vi "Load Action Core.vi"(8 "error in (no error)":errorcluster, 10 "config file in":T1, 11 "NI DMM in":refnum<class "NI DMM.lvclass">) -> (0 "error out":errorcluster, 2 "config file out":T1, 3 "NI DMM out":refnum<class "NI DMM.lvclass">)   [LabVIEW 2023, in "NI DMM.lvlib" / "NI DMM.lvclass"]
uses:
  NI DMM.lvclass
  <vilib>/Utility/config.llb/Config Data RefNum.ctl
  NI DMM.lvclass/NI DMM.ctl
  <vilib>/Utility/config.llb/NI_LVConfig.lvlib
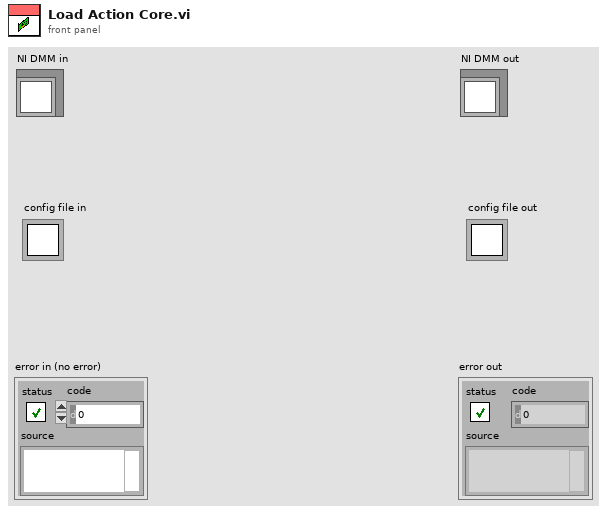
[diagram p1: front panel]
types:
  T1 = typedef "NI_LVConfig.lvlib/Config Data RefNum.ctl" = refnum<k1>
  T2 = cluster{"instrument_descriptor":refnum<k15>, "function":i32, "sampling_rate":dbl, "number_to_fetch":i32, "range":dbl}
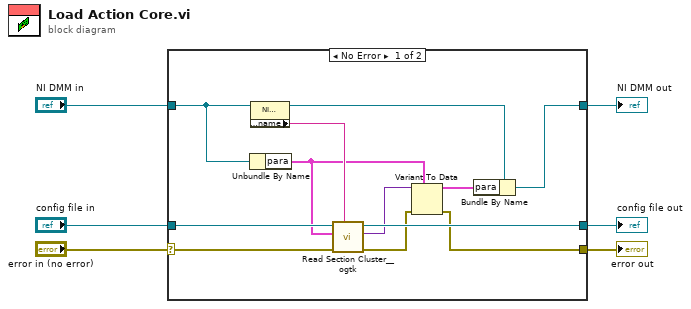
[diagram p0: block diagram]
diagram:
  n1 = case shown="No Error" "error in (no error)" {
    selector: "error in (no error)" -> [w18 w21]
    tunnel: [w12 w21] -> w5
    tunnel: "config file in" -> [w15 w20]
    tunnel: "NI DMM in" -> [w17 w19]
    tunnel: [w14 w20] -> w2
    tunnel: [w7 w19] -> w1
    frame No Error {
      n2 = Unbundle By Name(w17) -> ("para"=w11:T2)
      n3 = property class="NI DMM.lvclass"(reference=w17) -> (reference out=w9:refnum<class "NI DMM.lvclass">, "Accessor:name"=w16:string)  [unwired: 1 in, 1 out]
      n4 = call <userlib>:"Read Section Cluster__ogtk.vi"("section (optional)"=w16, "error in (no error)"=w18, "Section Formatted Cluster Type"=w11, "refnum"=w15) -> ("error out"=w13:errorcluster, "Section Formatted Cluster"=w10:variant, "dup refnum"=w14:T1)  [unwired: 3 in, 2 out]
      n5 = Variant To Data(error in=w13, type=w11, Variant=w10) -> (data=w8:T2, error out=w12:errorcluster)
      n6 = Bundle By Name(cluster=w9, "para"=w8) -> (w7:refnum<class "NI DMM.lvclass">)
    }
    frame Error {
    }
  }
  "error out" <- w5
  "NI DMM out" <- w1
  "config file out" <- w2
